vi "Example 1 - Write.vi"() -> ()   [LabVIEW 2021]
uses:
  SharedVariable_Bus/SharedVariable_Bus.lvclass
  C:/Program Files (x86)/National Instruments/LabVIEW 2021/vi.lib/TSA/Omni-Bus/Omni-Bus/Bus Access/Bus_Access.lvclass
  <vilib>/TSA/Omni-Bus/Omni-Bus/Omni_Bus.lvclass
  <vilib>/TSA/Omni-Bus/Omni-Bus/Support/Write/Write Boolean.vi
  <vilib>/TSA/Omni-Bus/Omni-Bus/Support/Write/Write DBL.vi
  <vilib>/TSA/Abstract Data Classes/Abs_Types/Boolean/Abs_Boolean.lvclass
  C:/Program Files (x86)/National Instruments/LabVIEW 2021/vi.lib/TSA/Abstract Data Classes/Abs_Types/Type/Abs_Type.lvclass
  <vilib>/TSA/Abstract Data Classes/Abs_Types/Double Float/Abs_Double Float.lvclass
  <vilib>/TSA/Omni-Bus/Omni-Bus/Support/FindVar.vi
panel:
  out "error out 2":errorcluster
  out "error out":errorcluster
  in  "stop":bool
  in  "Numeric":dbl
  in  "Boolean":bool
  out "DBL":dbl
  out "Bool":bool
  in  "Numeric Tag":string="ni.var.psp://localhost/SV Test/DBL"
  in  "Bool Tag":string="ni.var.psp://localhost/SV Test/Bool"
  out "Tags":string[](array[string])
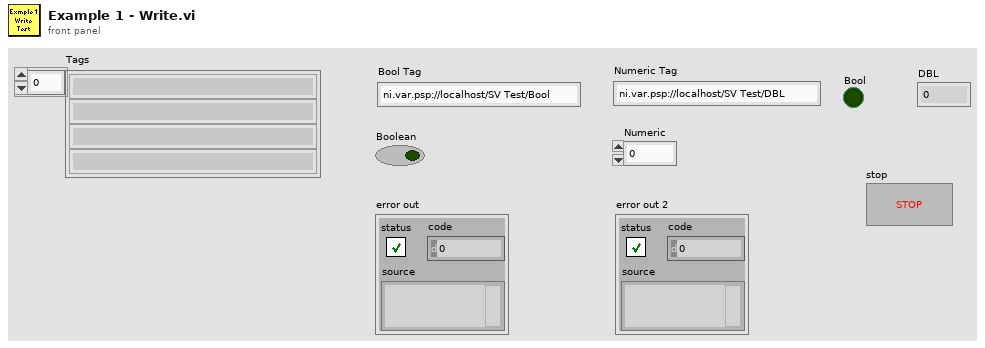
[diagram p1: front panel]
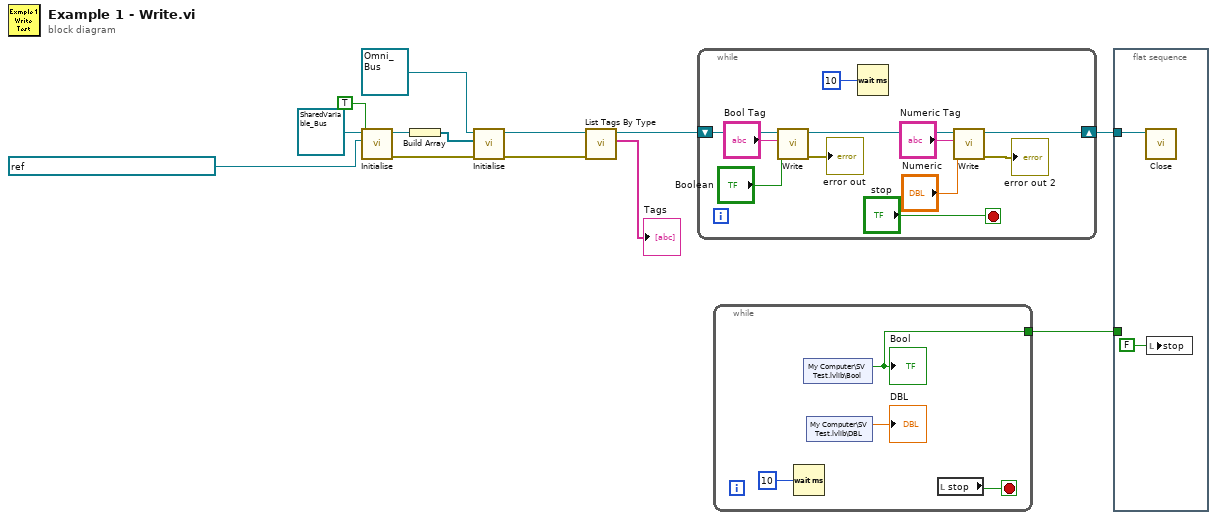
[diagram p0: block diagram]
diagram:
  n1 = call "Initialise.vi"("Include Container Name with Tag"=TRUE ("Add Container Name to Tag"), "SV Container"=refnum<k21> "ni.var.psp://my computer/SV Test" ("container refnum in"), "SharedVariable_Bus in"=refnum<class "SharedVariable_Bus.lvclass"> refnum) -> ("error out"=w11:errorcluster, "SharedVariable_Bus out"=w10:refnum<class "SharedVariable_Bus.lvclass">)  [unwired: 7 in]
  n2 = Build Array(w10) -> (w9:refnum<class "SharedVariable_Bus.lvclass">[])
  n3 = call-dynamic "Initialise.vi"("error in (no error)"=w11, "Bus Access"=w9, "Var Bus in"=refnum<class "Omni_Bus.lvclass"> refnum) -> ("error out"=w6:errorcluster, "Var Bus out"=w7:refnum<class "Omni_Bus.lvclass">)  [unwired: 7 in]
  n4 = call <vilib>:"List Tags By Type.vi"("error in (no error)"=w6, "Var Bus in"=w7) -> ("Tags"=→"Tags":string[], "Var Bus out"=w4:refnum<class "Omni_Bus.lvclass">)  [unwired: 6 in, 2 out]
  n5 = while {
    shift-right: [w22] -> w3
    shift-left: w4 -> [w24]
    stop <- "stop" stop-if-true
    n6 = call-poly <vilib>:"Write.vi"("Boolean"="Boolean", "Tag"="Bool Tag", "Omni_Bus in"=w24) -> ("error out"=→"error out":errorcluster, "Omni_Bus out"=w23:refnum<class "Omni_Bus.lvclass">)  [unwired: 7 in]
    n7 = Wait (ms)(milliseconds to wait=u32 10) -> ()  [unwired: 1 out]
    n8 = call-poly <vilib>:"Write.vi"("Numeric"="Numeric", "Tag"="Numeric Tag", "Omni_Bus in"=w23) -> ("error out"=→"error out 2":errorcluster, "Omni_Bus out"=w22:refnum<class "Omni_Bus.lvclass">)  [unwired: 7 in]
  }
  n9 = while {
    tunnel: [w25] -> w2
    stop <- w26 stop-if-true
    n10 = Wait (ms)(milliseconds to wait=u32 10) -> ()  [unwired: 1 out]
    n11 = shared-variable "My Computer\\SV Test.lvlib\\Bool"() -> (w25:bool)  [unwired: 1 in, 1 out]
    "Bool" <- w25
    n12 = shared-variable "My Computer\\SV Test.lvlib\\DBL"() -> (→"DBL":dbl)  [unwired: 1 in, 1 out]
    n13 = local read "stop"() -> (w26:bool)
  }
  n14 = flat-sequence {
    tunnel: w3 -> [w30]
    tunnel: w2 -> [_]
    frame #0 {
      n15 = call-dynamic "Close.vi"("Data in"=w30) -> ()  [unwired: 9 in, 2 out]
      n16 = local write "stop"(FALSE ("stop")) -> ()
    }
  }
